vi "Write dRA_ArcsPS.vi"(8 "error in (no error)":errorcluster, 10 "dRA_ArcsPS":dbl[unit] min=0.0 max=4.84813681109536e-05, 11 "DifftrackRADec in":refnum<class "DifftrackRADec.lvclass">) -> (0 "error out":errorcluster, 3 "DifftrackRADec out":refnum<class "DifftrackRADec.lvclass">)   [LabVIEW 2014, in "TCSDataDefinitions.lvlib" / "TCSCommand.lvlib" / "TargetConfiguration.lvlib" / "Target.lvlib" / "DifftrackRADec.lvclass"]
uses:
  DifftrackRADec.lvclass
  DifftrackRADec.lvclass/DifftrackRADec.ctl
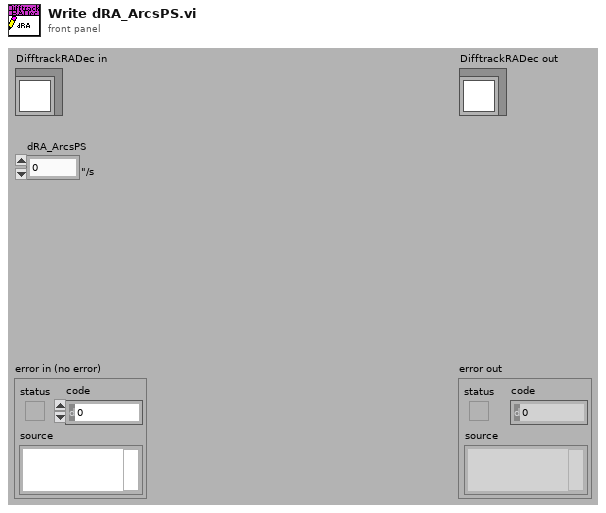
[diagram p1: front panel]
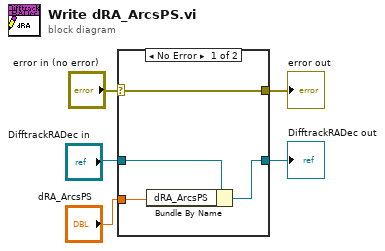
[diagram p0: block diagram]
diagram:
  n1 = case shown="No Error" "error in (no error)" {
    selector: "error in (no error)" -> [w9 w10]
    tunnel: [w9 w10] -> w4
    tunnel: [w7 w11] -> w2
    tunnel: "DifftrackRADec in" -> [w8 w11]
    tunnel: "dRA_ArcsPS" -> [w6 _]
    frame No Error {
      n2 = Bundle By Name(cluster=w8, "dRA_ArcsPS"=w6) -> (w7:refnum<class "DifftrackRADec.lvclass">)
    }
    frame Error {
    }
  }
  "error out" <- w4
  "DifftrackRADec out" <- w2
